vi "观察者模式DEMO.vi"() -> ()   [LabVIEW 2013]
uses:
  DAQ_class/DAQ.lvclass
  Display_class/Display.lvclass
  Save_class/Save.lvclass
  Subject_class/Subject.lvclass
  <vilib>/addons/_AddQ/G#Object/G#Object.lvclass
panel:
  out "# of objects killed":i32
  in  "停止":bool
  out "Output":string
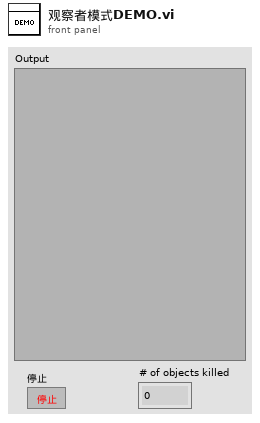
[diagram p1: front panel]
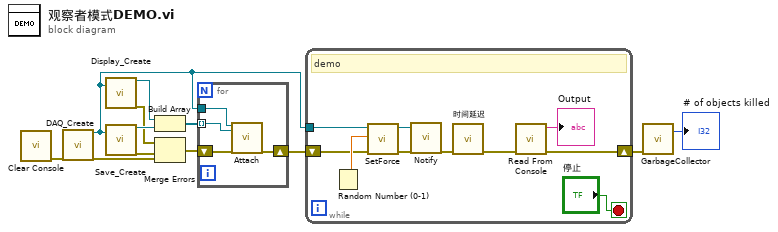
[diagram p0: block diagram]
diagram:
  n1 = call "Clear Console.vi"() -> ("error out"=w3:errorcluster)  [unwired: 11 in]
  n2 = call "DAQ_Create.vi"("error in (no error)"=w3) -> ("reference out"=w5:refnum<class "DAQ.lvclass">, "error out"=w7:errorcluster)  [unwired: 17 in]
  n3 = call "Display_Create.vi"("DAQ.lvclass"=w5) -> ("reference out"=w10:refnum<class "Display.lvclass">, "error out"=w9:errorcluster)  [unwired: 17 in]
  n4 = call "Save_Create.vi"("DAQ.lvclass"=w5) -> ("reference out"=w12:refnum<class "Save.lvclass">, "error out"=w8:errorcluster)  [unwired: 17 in]
  n5 = Build Array(w10, w12) -> (w11:refnum<class "ObServer.lvclass">[])
  n6 = Merge Errors(w9, w8, w7) -> (w6:errorcluster)
  n7 = for {
    tunnel: w11 -> [w16] mode=indexing
    tunnel: w5 -> [w15]
    shift-right: [w13] -> w4
    shift-left: w6 -> [w14]
    n8 = call "Attach.vi"("reference in"=w15, "ObServer.lvclass"=w16, "error in (no error)"=w14) -> ("error out"=w13:errorcluster)  [unwired: 15 in, 1 out]
  }
  n9 = while "While循环" {
    tunnel: w5 -> [w22]
    shift-right: [w19] -> w2
    shift-left: w4 -> [w25]
    stop <- "停止" stop-if-true
    # "demo"
    n10 = Random Number (0-1)() -> (number: 0 to 1=w26:dbl)
    n11 = call-dynamic "SetForce.vi"("error in (no error)"=w25, "Force"=w26, "reference in"=w22) -> ("error out"=w23:errorcluster, "reference out"=w24:refnum<class "DAQ.lvclass">)  [unwired: 7 in]
    n12 = call "Notify.vi"("reference in"=w24, "error in (no error)"=w23) -> ("error out"=w21:errorcluster)  [unwired: 16 in, 1 out]
    n13 = call "时间延迟"("error in (no error)"=w21) -> ("error out"=w20:errorcluster)  [unwired: 10 in]
    n14 = call "Read From Console.vi"("error in (no error)"=w20) -> ("error out"=w19:errorcluster, "Output"=→"Output":string)  [unwired: 9 in]
  }
  n15 = call <vilib>:"GarbageCollector.vi"("error in (no error)"=w2) -> ("# of objects killed"=→"# of objects killed":i32)  [unwired: 16 in, 2 out]
